vi "getSettings.vi"(8 "error in (no error)":errorcluster, 11 "ICCameraAcquisitor in":refnum<class "ICCameraAcquisitor.lvclass">) -> (0 "error out":errorcluster, 3 "ICCameraAcquisitor out":refnum<class "ICCameraAcquisitor.lvclass">)   [LabVIEW 2009, in "Hardware.lvlib" / "Channels.lvlib" / "ICCameraAcquisitor.lvclass"]
uses:
  ICCameraAcquisitor.lvclass
panel:
  out "Exposure Time":dbl
  out "Number of Images":dbl
  out "Gain":dbl
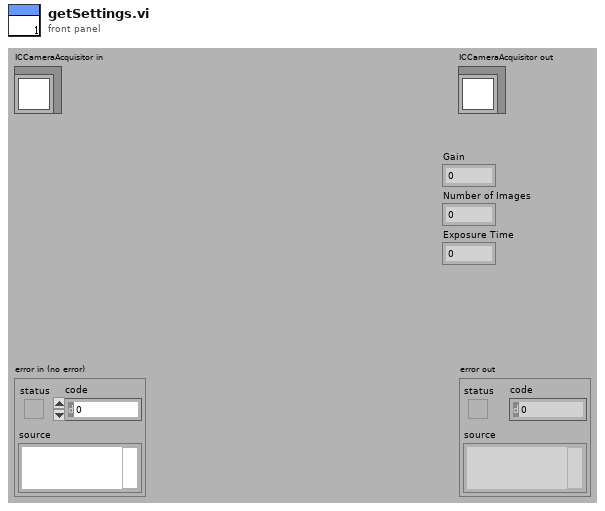
[diagram p1: front panel]
types:
  T1 = cluster{"Acquisition mode":dbl, "Readout Mode":dbl, "Gain":dbl}
  T2 = cluster{"shutter Open Time":dbl, "Shutter Close Time":dbl, "Exposure Time":dbl, " AccumulatedCycleTime":dbl, " KineticCycleTime":dbl, "Number of Accumulations":dbl, "Number in Kinetic Series ":dbl, "Shutter Mode":dbl}
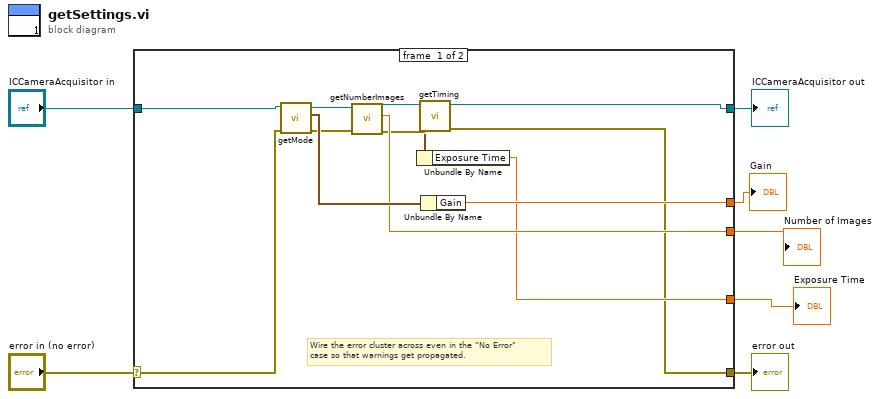
[diagram p0: block diagram]
diagram:
  n1 = case shown="No Error" "error in (no error)" {
    selector: "error in (no error)" -> [w8 w22]
    tunnel: [w9 w22] -> w6
    tunnel: [w10 w21] -> w4
    tunnel: "ICCameraAcquisitor in" -> [w20 w21]
    tunnel: [w18 _] -> w3
    tunnel: [w15 _] -> w2
    tunnel: [w11 _] -> w1
    frame #0 {
      # "Wire the error cluster across even in the \"No Error\"\ncase so that warnings get propagated."
      n2 = call-dynamic "getMode.vi"("error in (no error)"=w8, "CameraAcquisitor.lvclass in"=w20) -> ("error out"=w16:errorcluster, "Mode"=w19:T1, "CameraAcquisitor.lvclass out"=w17:refnum<class "ICCameraAcquisitor.lvclass">)  [unwired: 7 in]
      n3 = call-dynamic "getNumberImages.vi"("error in (no error)"=w16, "CameraAcquisitor.lvclass in"=w17) -> ("error out"=w13:errorcluster, "Number of Images"=w15:dbl, "CameraAcquisitor.lvclass out"=w14:refnum<class "ICCameraAcquisitor.lvclass">)  [unwired: 7 in]
      n4 = call-dynamic "getTiming.vi"("error in (no error)"=w13, "CameraAcquisitor.lvclass in"=w14) -> ("error out"=w9:errorcluster, "Timing"=w12:T2, "CameraAcquisitor.lvclass out"=w10:refnum<class "ICCameraAcquisitor.lvclass">)  [unwired: 7 in]
      n5 = Unbundle By Name(w12) -> ("Exposure Time"=w11:dbl)
      n6 = Unbundle By Name(w19) -> ("Gain"=w18:dbl)
    }
    frame #1 {
    }
  }
  "error out" <- w6
  "ICCameraAcquisitor out" <- w4
  "Gain" <- w3
  "Number of Images" <- w2
  "Exposure Time" <- w1
